vi "trivialhost.vi"() -> ()   [LabVIEW 2009]
panel:
  out "OUT":dbl
  in  "IN":dbl
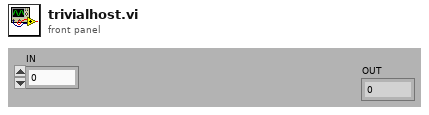
[diagram p1: front panel]
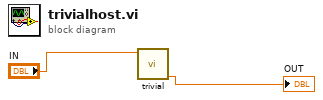
[diagram p0: block diagram]
diagram:
  n1 = call "trivial.vi"("IN"="IN") -> ("OUT"=→"OUT":dbl)  [unwired: 10 in]
